vi "M0203.vi"   [LabVIEW 2016]
uses:
  <vilib>/NXT/Block Support/NXT_InputPort.ctl
types:
  T1 = typedef "NXT_InputPort.ctl" = u32
  T2 = typedef "LVHSConnector.ctl" = refnum<class "BrickReference.lvclass">
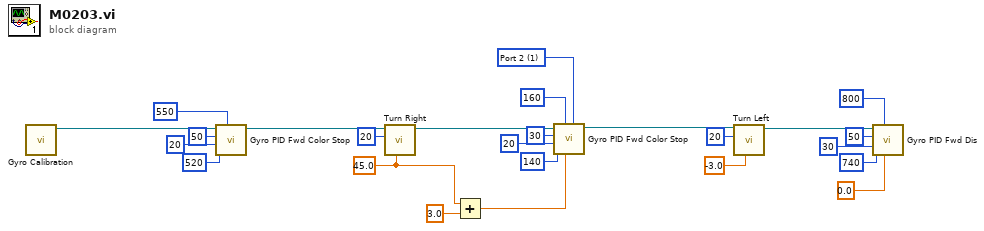
[diagram p0: block diagram]
diagram:
  w17 = T1 1 items=["Port 1", "Port 2", "Port 3", "Port 4"] ("Port")
  w12 = sgl 45.0 ("Turning angle")
  n1 = call "Gyro Calibration.vi"() -> ("NXT/EV3"=w25:T2)  [unwired: 7 in, 2 out]
  n2 = call "Gyro PID Fwd Color Stop.vi"("Threshold to Color"=550 ("Threshold to swtich"), "Threshold to slow"=520, "Min. speed"=20, "Max. speed"=50, "EV3 in"=w25) -> ("EV3 out"=w20:T2)  [unwired: 6 in]
  n3 = call "Turn Right.vi"("Turning angle"=w12, "Motor B (right)"=i8 20, "EV3 in"=w20) -> ("EV3 out"=w18:T2)  [unwired: 8 in]
  n4 = Add(x=w12, y=sgl 3.0) -> (x+y=w10:sgl)
  n5 = call "Gyro PID Fwd Color Stop.vi"("Port"=w17, "Target angle"=w10, "Threshold to Color"=160, "Threshold to slow"=140, "Min. speed"=20, "Max. speed"=30, "EV3 in"=w18) -> ("EV3 out"=w9:T2)  [unwired: 4 in]
  n6 = call "Turn Left.vi"("Turning angle"=sgl -3.0, "Motor B (right)"=i8 20, "EV3 in"=w9) -> ("EV3 out"=w6:T2)  [unwired: 8 in]
  n7 = call "Gyro PID Fwd Dis.vi"("Target angle"=sgl 0.0, "Threshold to stop"=800, "Threshold to slow"=740, "Min. speed"=30, "Max. speed"=50, "EV3 in"=w6) -> ()  [unwired: 5 in, 1 out]
